vi "read Txt Files.vi"(10 "file path (use dialog)":path) -> (1 "error out":errorcluster, 2 "number":T1)   [LabVIEW 2017] (continued)
Voltage¡G\t0.005524\nReal Periold(ms)¡G\t1\tEncoder Position(0.1mm)¡G\t0.000000\tVelocity(0.1mm0/s)¡G\t0.000000\tVoltage¡G\t-0.016754\nReal Periold(ms)¡G\t1\tEncoder Position(0.1mm)¡G\t0.000000\tVelocity(0.1mm0/s)¡G\t0.000000\tVoltage¡G\t-0.003723\nReal Periold(ms)¡G\t1\tEncoder Position(0.1mm)¡G\t0.000000\tVelocity(0.1mm0/s)¡G\t0.000000\tVoltage¡G\t0.012512\nReal Periold(ms)¡G\t1\tEncoder Position(0.1mm)¡G\t0.000000\tVelocity(0.1mm0/s)¡G\t0.000000\tVoltage¡G\t0.006775\nReal Periold(ms)¡G\t1\tEncoder Position(0.1mm)¡G\t0.000000\tVelocity(0.1mm0/s)¡G\t0.000000\tVoltage¡G\t-0.003082\nReal Periold(ms)¡G\t1\tEncoder Position(0.1mm)¡G\t0.000000\tVelocity(0.1mm0/s)¡G\t0.000000\tVoltage¡G\t-0.003387\nReal Periold(ms)¡G\t1\tEncoder Position(0.1mm)¡G\t0.000000\tVelocity(0.1mm0/s)¡G\t0.000000\tVoltage¡G\t0.005524\nReal Periold(ms)¡G\t1\tEncoder Position(0.1mm)¡G\t0.000000\tVelocity(0.1mm0/s)¡G\t0.000000\tVoltage¡G\t-0.001160\nReal Periold(ms)¡G\t1\tEncoder Position(0.1mm)¡G\t0.000000\tVelocity(0.1mm0/s)¡G\t0.000000\tVoltage¡G\t-0.001495\nReal Periold(ms)¡G\t1\tEncoder Position(0.1mm)¡G\t0.000000\tVelocity(0.1mm0/s)¡G\t0.000000\tVoltage¡G\t0.001678\nReal Periold(ms)¡G\t1\tEncoder Position(0.1mm)¡G\t0.000000\tVelocity(0.1mm0/s)¡G\t0.000000\tVoltage¡G\t-0.014221\nReal Periold(ms)¡G\t1\tEncoder Position(0.1mm)¡G\t0.000000\tVelocity(0.1mm0/s)¡G\t0.000000\tVoltage¡G\t-0.005005\nReal Periold(ms)¡G\t1\tEncoder Position(0.1mm)¡G\t0.000000\tVelocity(0.1mm0/s)¡G\t0.000000\tVoltage¡G\t0.003906\nReal Periold(ms)¡G\t1\tEncoder Position(0.1mm)¡G\t0.000000\tVelocity(0.1mm0/s)¡G\t0.000000\tVoltage¡G\t-0.000214\nReal Periold(ms)¡G\t1\tEncoder Position(0.1mm)¡G\t0.000000\tVelocity(0.1mm0/s)¡G\t0.000000\tVoltage¡G\t0.001678\nReal Periold(ms)¡G\t1\tEncoder Position(0.1mm)¡G\t0.000000\tVelocity(0.1mm0/s)¡G\t0.000000\tVoltage¡G\t-0.009766\nReal Periold(ms)¡G\t1\tEncoder Position(0.1mm)¡G\t0.000000\tVelocity(0.1mm0/s)¡G\t0.000000\tVoltage¡G\t-0.021240\nReal Periold(ms)¡G\t1\tEncoder Position(0.1mm)¡G\t0.000000\tVelocity(0.1mm0/s)¡G\t0.000000\tVoltage¡G\t0.002319\nReal Periold(ms)¡G\t1\tEncoder Position(0.1mm)¡G\t0.000000\tVelocity(0.1mm0/s)¡G\t0.000000\tVoltage¡G\t-0.000854\nReal Periold(ms)¡G\t1\tEncoder Position(0.1mm)¡G\t0.000000\tVelocity(0.1mm0/s)¡G\t0.000000\tVoltage¡G\t0.006470\nReal Periold(ms)¡G\t1\tEncoder Position(0.1mm)¡G\t0.000000\tVelocity(0.1mm0/s)¡G\t0.000000\tVoltage¡G\t-0.002777\nReal Periold(ms)¡G\t1\tEncoder Position(0.1mm)¡G\t0.000000\tVelocity(0.1mm0/s)¡G\t0.000000\tVoltage¡G\t-0.004028\nReal Periold(ms)¡G\t1\tEncoder Position(0.1mm)¡G\t0.000000\tVelocity(0.1mm0/s)¡G\t0.000000\tVoltage¡G\t-0.016144\nReal Periold(ms)¡G\t1\tEncoder Position(0.1mm)¡G\t0.000000\tVelocity(0.1mm0/s)¡G\t0.000000\tVoltage¡G\t0.004547\nReal Periold(ms)¡G\t1\tEncoder Position(0.1mm)¡G\t0.000000\tVelocity(0.1mm0/s)¡G\t0.000000\tVoltage¡G\t-0.010071\nReal Periold(ms)¡G\t1\tEncoder Position(0.1mm)¡G\t0.000000\tVelocity(0.1mm0/s)¡G\t0.000000\tVoltage¡G\t-0.008179\nReal Periold(ms)¡G\t1\tEncoder Position(0.1mm)¡G\t0.000000\tVelocity(0.1mm0/s)¡G\t0.000000\tVoltage¡G\t-0.011047\nReal Periold(ms)¡G\t1\tEncoder Position(0.1mm)¡G\t0.000000\tVelocity(0.1mm0/s)¡G\t0.000000\tVoltage¡G\t-0.005951\nReal Periold(ms)¡G\t1\tEncoder Position(0.1mm)¡G\t0.000000\tVelocity(0.1mm0/s)¡G\t0.000000\tVoltage¡G\t0.002960\nReal Periold(ms)¡G\t1\tEncoder Position(0.1mm)¡G\t0.000000\tVelocity(0.1mm0/s)¡G\t0.000000\tVoltage¡G\t0.002960\nReal Periold(ms)¡G\t1\tEncoder Position(0.1mm)¡G\t0.000000\tVelocity(0.1mm0/s)¡G\t0.000000\tVoltage¡G\t0.007751\nReal Periold(ms)¡G\t1\tEncoder Position(0.1mm)¡G\t0.000000\tVelocity(0.1mm0/s)¡G\t0.000000\tVoltage¡G\t-0.003387\nReal Periold(ms)¡G\t1\tEncoder Position(0.1mm)¡G\t0.000000\tVelocity(0.1mm0/s)¡G\t0.000000\tVoltage¡G\t-0.005615\nReal Periold(ms)¡G\t1\tEncoder Position(0.1mm)¡G\t0.000000\tVelocity(0.1mm0/s)¡G\t0.000000\tVoltage¡G\t-0.002136\nReal Periold(ms)¡G\t1\tEncoder Position(0.1mm)¡G\t0.000000\tVelocity(0.1mm0/s)¡G\t0.000000\tVoltage¡G\t-0.002777\nReal Periold(ms)¡G\t1\tEncoder Position(0.1mm)¡G\t0.000000\tVelocity(0.1mm0/s)¡G\t0.000000\tVoltage¡G\t-0.007843\nReal Periold(ms)¡G\t1\tEncoder Position(0.1mm)¡G\t0.000000\tVelocity(0.1mm0/s)¡G\t0.000000\tVoltage¡G\t0.000732\nReal Periold(ms)¡G\t1\tEncoder Position(0.1mm)¡G\t0.000000\tVelocity(0.1mm0/s)¡G\t0.000000\tVoltage¡G\t-0.001495\nReal Periold(ms)¡G\t1\tEncoder Position(0.1mm)¡G\t0.000000\tVelocity(0.1mm0/s)¡G\t0.000000\tVoltage¡G\t-0.008179\nReal Periold(ms)¡G\t1\tEncoder Position(0.1mm)¡G\t0.000000\tVelocity(0.1mm0/s)¡G\t0.000000\tVoltage¡G\t-0.010406\nReal Periold(ms)¡G\t1\tEncoder Position(0.1mm)¡G\t0.000000\tVelocity(0.1mm0/s)¡G\t0.000000\tVoltage¡G\t-0.003723\nReal Periold(ms)¡G\t1\tEncoder Position(0.1mm)¡G\t0.000000\tVelocity(0.1mm0/s)¡G\t0.000000\tVoltage¡G\t0.002319\nReal Periold(ms)¡G\t1\tEncoder Position(0.1mm)¡G\t0.000000\tVelocity(0.1mm0/s)¡G\t0.000000\tVoltage¡G\t-0.001495\nReal Periold(ms)¡G\t1\tEncoder Position(0.1mm)¡G\t0.000000\tVelocity(0.1mm0/s)¡G\t0.000000\tVoltage¡G\t0.004242\nReal Periold(ms)¡G\t1\tEncoder Position(0.1mm)¡G\t0.000000\tVelocity(0.1mm0/s)¡G\t0.000000\tVoltage¡G\t0.011566\nReal Periold(ms)¡G\t1\tEncoder Position(0.1mm)¡G\t0.000000\tVelocity(0.1mm0/s)¡G\t0.000000\tVoltage¡G\t-0.000214\nReal Periold(ms)¡G\t1\tEncoder Position(0.1mm)¡G\t0.000000\tVelocity(0.1mm0/s)¡G\t0.000000\tVoltage¡G\t0.004242\nReal Periold(ms)¡G\t1\tEncoder Position(0.1mm)¡G\t0.000000\tVelocity(0.1mm0/s)¡G\t0.000000\tVoltage¡G\t-0.009125\nReal Periold(ms)¡G\t1\tEncoder Position(0.1mm)¡G\t0.000000\tVelocity(0.1mm0/s)¡G\t0.000000\tVoltage¡G\t-0.000854\nReal Periold(ms)¡G\t1\tEncoder Position(0.1mm)¡G\t0.000000\tVelocity(0.1mm0/s)¡G\t0.000000\tVoltage¡G\t-0.004669\nReal Periold(ms)¡G\t1\tEncoder Position(0.1mm)¡G\t0.000000\tVelocity(0.1mm0/s)¡G\t0.000000\tVoltage¡G\t0.005829\nReal Periold(ms)¡G\t1\tEncoder Position(0.1mm)¡G\t0.000000\tVelocity(0.1mm0/s)¡G\t0.000000\tVoltage¡G\t-0.013580\nReal Periold(ms)¡G\t1\tEncoder Position(0.1mm)¡G\t0.000000\tVelocity(0.1mm0/s)¡G\t0.000000\tVoltage¡G\t-0.005951\nReal Periold(ms)¡G\t1\tEncoder Position(0.1mm)¡G\t0.000000\tVelocity(0.1mm0/s)¡G\t0.000000\tVoltage¡G\t-0.002777\nReal Periold(ms)¡G\t1\tEncoder Position(0.1mm)¡G\t0.000000\tVelocity(0.1mm0/s)¡G\t0.000000\tVoltage¡G\t0.006470\nReal Periold(ms)¡G\t1\tEncoder Position(0.1mm)¡G\t0.000000\tVelocity(0.1mm0/s)¡G\t0.000000\tVoltage¡G\t0.000427\nReal Periold(ms)¡G\t1\tEncoder Position(0.1mm)¡G\t0.000000\tVelocity(0.1mm0/s)¡G\t0.000000\tVoltage¡G\t0.008362\nReal Periold(ms)¡G\t1\tEncoder Position(0.1mm)¡G\t0.000000\tVelocity(0.1mm0/s)¡G\t0.000000\tVoltage¡G\t0.000092\nReal Periold(ms)¡G\t1\tEncoder Position(0.1mm)¡G\t0.000000\tVelocity(0.1mm0/s)¡G\t0.000000\tVoltage¡G\t-0.004028\nReal Periold(ms)¡G\t1\tEncoder Position(0.1mm)¡G\t0.000000\tVelocity(0.1mm0/s)¡G\t0.000000\tVoltage¡G\t-0.004364\nReal Periold(ms)¡G\t1\tEncoder Position(0.1mm)¡G\t0.000000\tVelocity(0.1mm0/s)¡G\t0.000000\tVoltage¡G\t0.007111\nReal Periold(ms)¡G\t1\tEncoder Position(0.1mm)¡G\t0.000000\tVelocity(0.1mm0/s)¡G\t0.000000\tVoltage¡G\t-0.013916\nReal Periold(ms)¡G\t1\tEncoder Position(0.1mm)¡G\t0.000000\tVelocity(0.1mm0/s)¡G\t0.000000\tVoltage¡G\t0.000732\nReal Periold(ms)¡G\t1\tEncoder Position(0.1mm)¡G\t0.000000\tVelocity(0.1mm0/s)¡G\t0.000000\tVoltage¡G\t-0.009766\nReal Periold(ms)¡G\t1\tEncoder Position(0.1mm)¡G\t0.000000\tVelocity(0.1mm0/s)¡G\t0.000000\tVoltage¡G\t0.000092\nReal Periold(ms)¡G\t1\tEncoder Position(0.1mm)¡G\t0.000000\tVelocity(0.1mm0/s)¡G\t0.000000\tVoltage¡G\t0.002319\nReal Periold(ms)¡G\t1\tEncoder Position(0.1mm)¡G\t0.000000\tVelocity(0.1mm0/s)¡G\t0.000000\tVoltage¡G\t-0.005005\nReal Periold(ms)¡G\t1\tEncoder Position(0.1mm)¡G\t0.000000\tVelocity(0.1mm0/s)¡G\t0.000000\tVoltage¡G\t0.009003\nReal Periold(ms)¡G\t1\tEncoder Position(0.1mm)¡G\t0.000000\tVelocity(0.1mm0/s)¡G\t0.000000\tVoltage¡G\t0.014099\nReal Periold(ms)¡G\t1\tEncoder Position(0.1mm)¡G\t0.000000\tVelocity(0.1mm0/s)¡G\t0.000000\tVoltage¡G\t0.002960\nReal Periold(ms)¡G\t1\tEncoder Position(0.1mm)¡G\t0.000000\tVelocity(0.1mm0/s)¡G\t0.000000\tVoltage¡G\t0.000732\nReal Periold(ms)¡G\t1\tEncoder Position(0.1mm)¡G\t0.000000\tVelocity(0.1mm0/s)¡G\t0.000000\tVoltage¡G\t-0.005310\nReal Periold(ms)¡G\t1\tEncoder Position(0.1mm)¡G\t0.000000\tVelocity(0.1mm0/s)¡G\t0.000000\tVoltage¡G\t0.003906\nReal Periold(ms)¡G\t1\tEncoder Position(0.1mm)¡G\t0.000000\tVelocity(0.1mm0/s)¡G\t0.000000\tVoltage¡G\t-0.034271\nReal Periold(ms)¡G\t1\tEncoder Position(0.1mm)¡G\t0.000000\tVelocity(0.1mm0/s)¡G\t0.000000\tVoltage¡G\t-0.012634\nReal Periold(ms)¡G\t1\tEncoder Position(0.1mm)¡G\t0.000000\tVelocity(0.1mm0/s)¡G\t0.000000\tVoltage¡G\t-0.002136\nReal Periold(ms)¡G\t1\tEncoder Position(0.1mm)¡G\t0.000000\tVelocity(0.1mm0/s)¡G\t0.000000\tVoltage¡G\t0.009644\nReal Periold(ms)¡G\t1\tEncoder Position(0.1mm)¡G\t0.000000\tVelocity(0.1mm0/s)¡G\t0.000000\tVoltage¡G\t0.000092\nReal Periold(ms)¡G\t1\tEncoder Position(0.1mm)¡G\t0.000000\tVelocity(0.1mm0/s)¡G\t0.000000\tVoltage¡G\t0.000427\nReal Periold(ms)¡G\t1\tEncoder Position(0.1mm)¡G\t0.000000\tVelocity(0.1mm0/s)¡G\t0.000000\tVoltage¡G\t-0.002441\nReal Periold(ms)¡G\t1\tEncoder Position(0.1mm)¡G\t0.000000\tVelocity(0.1mm0/s)¡G\t0.000000\tVoltage¡G\t-0.006256\nReal Periold(ms)¡G\t1\tEncoder Position(0.1mm)¡G\t0.000000\tVelocity(0.1mm0/s)¡G\t0.000000\tVoltage¡G\t0.007751\nReal Periold(ms)¡G\t1\tEncoder Position(0.1mm)¡G\t0.000000\tVelocity(0.1mm0/s)¡G\t0.000000\tVoltage¡G\t0.000092\nReal Periold(ms)¡G\t1\tEncoder Position(0.1mm)¡G\t0.000000\tVelocity(0.1mm0/s)¡G\t0.000000\tVoltage¡G\t0.008698\nReal Periold(ms)¡G\t1\tEncoder Position(0.1mm)¡G\t0.000000\tVelocity(0.1mm0/s)¡G\t0.000000\tVoltage¡G\t0.010590\nReal Periold(ms)¡G\t1\tEncoder Position(0.1mm)¡G\t0.000000\tVelocity(0.1mm0/s)¡G\t0.000000\tVoltage¡G\t-0.002441\nReal Periold(ms)¡G\t1\tEncoder Position(0.1mm)¡G\t0.000000\tVelocity(0.1mm0/s)¡G\t0.000000\tVoltage¡G\t-0.008484\nReal Periold(ms)¡G\t1\tEncoder Position(0.1mm)¡G\t0.000000\tVelocity(0.1mm0/s)¡G\t0.000000\tVoltage¡G\t-0.001801\nReal Periold(ms)¡G\t1\tEncoder Position(0.1mm)¡G\t0.000000\tVelocity(0.1mm0/s)¡G\t0.000000\tVoltage¡G\t0.001373\nReal Periold(ms)¡G\t1\tEncoder Position(0.1mm)¡G\t0.000000\tVelocity(0.1mm0/s)¡G\t0.000000\tVoltage¡G\t-0.011993\nReal Periold(ms)¡G\t1\tEncoder Position(0.1mm)¡G\t0.000000\tVelocity(0.1mm0/s)¡G\t0.000000\tVoltage¡G\t-0.005615\nReal Periold(ms)¡G\t1\tEncoder Position(0.1mm)¡G\t0.000000\tVelocity(0.1mm0/s)¡G\t0.000000\tVoltage¡G\t0.014740\nReal Periold(ms)¡G\t1\tEncoder Position(0.1mm)¡G\t0.000000\tVelocity(0.1mm0/s)¡G\t0.000000\tVoltage¡G\t-0.000214\nReal Periold(ms)¡G\t1\tEncoder Position(0.1mm)¡G\t0.000000\tVelocity(0.1mm0/s)¡G\t0.000000\tVoltage¡G\t0.009979\nReal Periold(ms)¡G\t1\tEncoder Position(0.1mm)¡G\t0.000000\tVelocity(0.1mm0/s)¡G\t0.000000\tVoltage¡G\t-0.002441\nReal Periold(ms)¡G\t1\tEncoder Position(0.1mm)¡G\t0.000000\tVelocity(0.1mm0/s)¡G\t0.000000\tVoltage¡G\t-0.005005\nReal Periold(ms)¡G\t1\tEncoder Position(0.1mm)¡G\t0.000000\tVelocity(0.1mm0/s)¡G\t0.000000\tVoltage¡G\t0.003601\nReal Periold(ms)¡G\t1\tEncoder Position(0.1mm)¡G\t0.000000\tVelocity(0.1mm0/s)¡G\t0.000000\tVoltage¡G\t0.002960\nReal Periold(ms)¡G\t1\tEncoder Position(0.1mm)¡G\t0.000000\tVelocity(0.1mm0/s)¡G\t0.000000\tVoltage¡G\t0.003601\nReal Periold(ms)¡G\t1\tEncoder Position(0.1mm)¡G\t0.000000\tVelocity(0.1mm0/s)¡G\t0.000000\tVoltage¡G\t-0.007843\nReal Periold(ms)¡G\t1\tEncoder Position(0.1mm)¡G\t0.000000\tVelocity(0.1mm0/s)¡G\t0.000000\tVoltage¡G\t-0.001495\nReal Periold(ms)¡G\t1\tEncoder Position(0.1mm)¡G\t0.000000\tVelocity(0.1mm0/s)¡G\t0.000000\tVoltage¡G\t-0.001495\nReal Periold(ms)¡G\t1\tEncoder Position(0.1mm)¡G\t0.000000\tVelocity(0.1mm0/s)¡G\t0.000000\tVoltage¡G\t0.002319\nReal Periold(ms)¡G\t1\tEncoder Position(0.1mm)¡G\t0.000000\tVelocity(0.1mm0/s)¡G\t0.000000\tVoltage¡G\t0.006775\nReal Periold(ms)¡G\t1\tEncoder Position(0.1mm)¡G\t0.000000\tVelocity(0.1mm0/s)¡G\t0.000000\tVoltage¡G\t0.000092\nReal Periold(ms)¡G\t1\tEncoder Position(0.1mm)¡G\t0.000000\tVelocity(0.1mm0/s)¡G\t0.000000\tVoltage¡G\t0.006134\nReal Periold(ms)¡G\t1\tEncoder Position(0.1mm)¡G\t0.000000\tVelocity(0.1mm0/s)¡G\t0.000000\tVoltage¡G\t0.003906\nReal Periold(ms)¡G\t1\tEncoder Position(0.1mm)¡G\t0.000000\tVelocity(0.1mm0/s)¡G\t0.000000\tVoltage¡G\t0.004883\nReal Periold(ms)¡G\t1\tEncoder Position(0.1mm)¡G\t0.000000\tVelocity(0.1mm0/s)¡G\t0.000000\tVoltage¡G\t-0.002777\nReal Periold(ms)¡G\t1\tEncoder Position(0.1mm)¡G\t0.000000\tVelocity(0.1mm0/s)¡G\t0.000000\tVoltage¡G\t-0.007538\nReal Periold(ms)¡G\t1\tEncoder Position(0.1mm)¡G\t0.000000\tVelocity(0.1mm0/s)¡G\t0.000000\tVoltage¡G\t-0.003387\nReal Periold(ms)¡G\t1\tEncoder Position(0.1mm)¡G\t0.000000\tVelocity(0.1mm0/s)¡G\t0.000000\tVoltage¡G\t-0.014526\nReal Periold(ms)¡G\t1\tEncoder Position(0.1mm)¡G\t0.000000\tVelocity(0.1mm0/s)¡G\t0.000000\tVoltage¡G\t-0.004364\nReal Periold(ms)¡G\t1\tEncoder Position(0.1mm)¡G\t0.000000\tVelocity(0.1mm0/s)¡G\t0.000000\tVoltage¡G\t-0.000549\nReal Periold(ms)¡G\t1\tEncoder Position(0.1mm)¡G\t0.000000\tVelocity(0.1mm0/s)¡G\t0.000000\tVoltage¡G\t0.003296\nReal Periold(ms)¡G\t1\tEncoder Position(0.1mm)¡G\t0.000000\tVelocity(0.1mm0/s)¡G\t0.000000\tVoltage¡G\t-0.004028\nReal Periold(ms)¡G\t1\tEncoder Position(0.1mm)¡G\t0.000000\tVelocity(0.1mm0/s)¡G\t0.000000\tVoltage¡G\t0.002960\nReal Periold(ms)¡G\t1\tEncoder Position(0.1mm)¡G\t0.000000\tVelocity(0.1mm0/s)¡G\t0.000000\tVoltage¡G\t-0.006256\nReal Periold(ms)¡G\t1\tEncoder Position(0.1mm)¡G\t0.000000\tVelocity(0.1mm0/s)¡G\t0.000000\tVoltage¡G\t0.004242\nReal Periold(ms)¡G\t1\tEncoder Position(0.1mm)¡G\t0.000000\tVelocity(0.1mm0/s)¡G\t0.000000\tVoltage¡G\t-0.013916\nReal Periold(ms)¡G\t1\tEncoder Position(0.1mm)¡G\t0.000000\tVelocity(0.1mm0/s)¡G\t0.000000\tVoltage¡G\t0.005188\nReal Periold(ms)¡G\t1\tEncoder Position(0.1mm)¡G\t0.000000\tVelocity(0.1mm0/s)¡G\t0.000000\tVoltage¡G\t-0.015808\nReal Periold(ms)¡G\t1\tEncoder Position(0.1mm)¡G\t0.000000\tVelocity(0.1mm0/s)¡G\t0.000000\tVoltage¡G\t-0.007843\nReal Periold(ms)¡G\t1\tEncoder Position(0.1mm)¡G\t0.000000\tVelocity(0.1mm0/s)¡G\t0.000000\tVoltage¡G\t-0.005310\nReal Periold(ms)¡G\t1\tEncoder Position(0.1mm)¡G\t0.000000\tVelocity(0.1mm0/s)¡G\t0.000000\tVoltage¡G\t0.002960\nReal Periold(ms)¡G\t1\tEncoder Position(0.1mm)¡G\t0.000000\tVelocity(0.1mm0/s)¡G\t0.000000\tVoltage¡G\t-0.006256\nReal Periold(ms)¡G\t1\tEncoder Position(0.1mm)¡G\t0.000000\tVelocity(0.1mm0/s)¡G\t0.000000\tVoltage¡G\t0.001678\nReal Periold(ms)¡G\t1\tEncoder Position(0.1mm)¡G\t0.000000\tVelocity(0.1mm0/s)¡G\t0.000000\tVoltage¡G\t-0.013916\nReal Periold(ms)¡G\t1\tEncoder Position(0.1mm)¡G\t0.000000\tVelocity(0.1mm0/s)¡G\t0.000000\tVoltage¡G\t0.007751\nReal Periold(ms)¡G\t1\tEncoder Position(0.1mm)¡G\t0.000000\tVelocity(0.1mm0/s)¡G\t0.000000\tVoltage¡G\t0.009338\nReal Periold(ms)¡G\t1\tEncoder Position(0.1mm)¡G\t0.000000\tVelocity(0.1mm0/s)¡G\t0.000000\tVoltage¡G\t-0.002136\nReal Periold(ms)¡G\t1\tEncoder Position(0.1mm)¡G\t0.000000\tVelocity(0.1mm0/s)¡G\t0.000000\tVoltage¡G\t0.002014\nReal Periold(ms)¡G\t1\tEncoder Position(0.1mm)¡G\t0.000000\tVelocity(0.1mm0/s)¡G\t0.000000\tVoltage¡G\t0.002319\nReal Periold(ms)¡G\t1\tEncoder Position(0.1mm)¡G\t0.000000\tVelocity(0.1mm0/s)¡G\t0.000000\tVoltage¡G\t-0.009125\nReal Periold(ms)¡G\t1\tEncoder Position(0.1mm)¡G\t0.000000\tVelocity(0.1mm0/s)¡G\t0.000000\tVoltage¡G\t0.001068\nReal Periold(ms)¡G\t1\tEncoder Position(0.1mm)¡G\t0.000000\tVelocity(0.1mm0/s)¡G\t0.000000\tVoltage¡G\t-0.011993\nReal Periold(ms)¡G\t1\tEncoder Position(0.1mm)¡G\t0.000000\tVelocity(0.1mm0/s)¡G\t0.000000\tVoltage¡G\t0.006470\nReal Periold(ms)¡G\t1\tEncoder Position(0.1mm)¡G\t0.000000\tVelocity(0.1mm0/s)¡G\t0.000000\tVoltage¡G\t-0.002136\nReal Periold(ms)¡G\t1\tEncoder Position(0.1mm)¡G\t0.000000\tVelocity(0.1mm0/s)¡G\t0.000000\tVoltage¡G\t-0.006592\nReal Periold(ms)¡G\t1\tEncoder Position(0.1mm)¡G\t0.000000\tVelocity(0.1mm0/s)¡G\t0.000000\tVoltage¡G\t-0.004364\nReal Periold(ms)¡G\t1\tEncoder Position(0.1mm)¡G\t0.000000\tVelocity(0.1mm0/s)¡G\t0.000000\tVoltage¡G\t0.000732\nReal Periold(ms)¡G\t1\tEncoder Position(0.1mm)¡G\t0.000000\tVelocity(0.1mm0/s)¡G\t0.000000\tVoltage¡G\t-0.012299\nReal Periold(ms)¡G\t1\tEncoder Position(0.1mm)¡G\t0.000000\tVelocity(0.1mm0/s)¡G\t0.000000\tVoltage¡G\t-0.000549\nReal Periold(ms)¡G\t1\tEncoder Position(0.1mm)¡G\t0.000000\tVelocity(0.1mm0/s)¡G\t0.000000\tVoltage¡G\t-0.006256\nReal Periold(ms)¡G\t1\tEncoder Position(0.1mm)¡G\t0.000000\tVelocity(0.1mm0/s)¡G\t0.000000\tVoltage¡G\t0.001373\nReal Periold(ms)¡G\t1\tEncoder Position(0.1mm)¡G\t0.000000\tVelocity(0.1mm0/s)¡G\t0.000000\tVoltage¡G\t0.004883\nReal Periold(ms)¡G\t1\tEncoder Position(0.1mm)¡G\t0.000000\tVelocity(0.1mm0/s)¡G\t0.000000\tVoltage¡G\t0.006134\nReal Periold(ms)¡G\t1\tEncoder Position(0.1mm)¡G\t0.000000\tVelocity(0.1mm0/s)¡G\t0.000000\tVoltage¡G\t-0.005615\nReal Periold(ms)¡G\t1\tEncoder Position(0.1mm)¡G\t0.000000\tVelocity(0.1mm0/s)¡G\t0.000000\tVoltage¡G\t0.003296\nReal Periold(ms)¡G\t1\tEncoder Position(0.1mm)¡G\t0.000000\tVelocity(0.1mm0/s)¡G\t0.000000\tVoltage¡G\t-0.003387\nReal Periold(ms)¡G\t1\tEncoder Position(0.1mm)¡G\t0.000000\tVelocity(0.1mm0/s)¡G\t0.000000\tVoltage¡G\t-0.012939\nReal Periold(ms)¡G\t1\tEncoder Position(0.1mm)¡G\t0.000000\tVelocity(0.1mm0/s)¡G\t0.000000\tVoltage¡G\t0.014740\nReal Periold(ms)¡G\t1\tEncoder Position(0.1mm)¡G\t0.000000\tVelocity(0.1mm0/s)¡G\t0.000000\tVoltage¡G\t-0.008179\nReal Periold(ms)¡G\t1\tEncoder Position(0.1mm)¡G\t0.000000\tVelocity(0.1mm0/s)¡G\t0.000000\tVoltage¡G\t-0.002441\nReal Periold(ms)¡G\t1\tEncoder Position(0.1mm)¡G\t0.000000\tVelocity(0.1mm0/s)¡G\t0.000000\tVoltage¡G\t-0.004364\nReal Periold(ms)¡G\t1\tEncoder Position(0.1mm)¡G\t0.000000\tVelocity(0.1mm0/s)¡G\t0.000000\tVoltage¡G\t0.002319\nReal Periold(ms)¡G\t1\tEncoder Position(0.1mm)¡G\t0.000000\tVelocity(0.1mm0/s)¡G\t0.000000\tVoltage¡G\t-0.003723\nReal Periold(ms)¡G\t1\tEncoder Position(0.1mm)¡G\t0.000000\tVelocity(0.1mm0/s)¡G\t0.000000\tVoltage¡G\t0.018890\nReal Periold(ms)¡G\t1\tEncoder Position(0.1mm)¡G\t0.000000\tVelocity(0.1mm0/s)¡G\t0.000000\tVoltage¡G\t0.007111\nReal Periold(ms)¡G\t1\tEncoder Position(0.1mm)¡G\t0.000000\tVelocity(0.1mm0/s)¡G\t0.000000\tVoltage¡G\t0.020782\nReal Periold(ms)¡G\t1\tEncoder Position(0.1mm)¡G\t0.000000\tVelocity(0.1mm0/s)¡G\t0.000000\tVoltage¡G\t-0.002136\nReal Periold(ms)¡G\t1\tEncoder Position(0.1mm)¡G\t0.000000\tVelocity(0.1mm0/s)¡G\t0.000000\tVoltage¡G\t0.003296\nReal Periold(ms)¡G\t1\tEncoder Position(0.1mm)¡G\t0.000000\tVelocity(0.1mm0/s)¡G\t0.000000\tVoltage¡G\t-0.010406\nReal Periold(ms)¡G\t1\tEncoder Position(0.1mm)¡G\t0.000000\tVelocity(0.1mm0/s)¡G\t0.000000\tVoltage¡G\t0.000092\nReal Periold(ms)¡G\t1\tEncoder Position(0.1mm)¡G\t0.000000\tVelocity(0.1mm0/s)¡G\t0.000000\tVoltage¡G\t-0.021240\nReal Periold(ms)¡G\t1\tEncoder Position(0.1mm)¡G\t0.000000\tVelocity(0.1mm0/s)¡G\t0.000000\tVoltage¡G\t-0.017731\nReal Periold(ms)¡G\t1\tEncoder Position(0.1mm)¡G\t0.000000\tVelocity(0.1mm0/s)¡G\t0.000000\tVoltage¡G\t-0.013275\nReal Periold(ms)¡G\t1\tEncoder Position(0.1mm)¡G\t0.000000\tVelocity(0.1mm0/s)¡G\t0.000000\tVoltage¡G\t-0.000214\nReal Periold(ms)¡G\t1\tEncoder Position(0.1mm)¡G\t0.000000\tVelocity(0.1mm0/s)¡G\t0.000000\tVoltage¡G\t-0.010071\nReal Periold(ms)¡G\t1\tEncoder Position(0.1mm)¡G\t0.000000\tVelocity(0.1mm0/s)¡G\t0.000000\tVoltage¡G\t-0.008179\nReal Periold(ms)¡G\t1\tEncoder Position(0.1mm)¡G\t0.000000\tVelocity(0.1mm0/s)¡G\t0.000000\tVoltage¡G\t-0.005615\nReal Periold(ms)¡G\t1\tEncoder Position(0.1mm)¡G\t0.000000\tVelocity(0.1mm0/s)¡G\t0.000000\tVoltage¡G\t-0.003723\nReal Periold(ms)¡G\t1\tEncoder Position(0.1mm)¡G\t0.000000\tVelocity(0.1mm0/s)¡G\t0.000000\tVoltage¡G\t-0.001160\nReal Periold(ms)¡G\t1\tEncoder Position(0.1mm)¡G\t0.000000\tVelocity(0.1mm0/s)¡G\t0.000000\tVoltage¡G\t0.003906\nReal Periold(ms)¡G\t1\tEncoder Position(0.1mm)¡G\t0.000000\tVelocity(0.1mm0/s)¡G\t0.000000\tVoltage¡G\t0.007111\nReal Periold(ms)¡G\t1\tEncoder Position(0.1mm)¡G\t0.000000\tVelocity(0.1mm0/s)¡G\t0.000000\tVoltage¡G\t-0.003082\nReal Periold(ms)¡G\t1\tEncoder Position(0.1mm)¡G\t0.000000\tVelocity(0.1mm0/s)¡G\t0.000000\tVoltage¡G\t-0.014221\nReal Periold(ms)¡G\t1\tEncoder Position(0.1mm)¡G\t0.000000\tVelocity(0.1mm0/s)¡G\t0.000000\tVoltage¡G\t-0.004364\nReal Periold(ms)¡G\t1\tEncoder Position(0.1mm)¡G\t0.000000\tVelocity(0.1mm0/s)¡G\t0.000000\tVoltage¡G\t0.000732\nReal Periold(ms)¡G\t1\tEncoder Position(0.1mm)¡G\t0.000000\tVelocity(0.1mm0/s)¡G\t0.000000\tVoltage¡G\t-0.016754\nReal Periold(ms)¡G\t1\tEncoder Position(0.1mm)¡G\t0.000000\tVelocity(0.1mm0/s)¡G\t0.000000\tVoltage¡G\t-0.014526\nReal Periold(ms)¡G\t1\tEncoder Position(0.1mm)¡G\t0.000000\tVelocity(0.1mm0/s)¡G\t0.000000\tVoltage¡G\t-0.012939\nReal Periold(ms)¡G\t1\tEncoder Position(0.1mm)¡G\t0.000000\tVelocity(0.1mm0/s)¡G\t0.000000\tVoltage¡G\t0.011566\nReal Periold(ms)¡G\t1\tEncoder Position(0.1mm)¡G\t0.000000\tVelocity(0.1mm0/s)¡G\t0.000000\tVoltage¡G\t0.017273\nReal Periold(ms)¡G\t1\tEncoder Position(0.1mm)¡G\t0.000000\tVelocity(0.1mm0/s)¡G\t0.000000\tVoltage¡G\t-0.004028\nReal Periold(ms)¡G\t1\tEncoder Position(0.1mm)¡G\t0.000000\tVelocity(0.1mm0/s)¡G\t0.000000\tVoltage¡G\t-0.006256\nReal Periold(ms)¡G\t1\tEncoder Position(0.1mm)¡G\t0.000000\tVelocity(0.1mm0/s)¡G\t0.000000\tVoltage¡G\t-0.004364\nReal Periold(ms)¡G\t1\tEncoder Position(0.1mm)¡G\t0.000000\tVelocity(0.1mm0/s)¡G\t0.000000\tVoltage¡G\t-0.011993\nReal Periold(ms)¡G\t1\tEncoder Position(0.1mm)¡G\t0.000000\tVelocity(0.1mm0/s)¡G\t0.000000\tVoltage¡G\t0.001373\nReal Periold(ms)¡G\t1\tEncoder Position(0.1mm)¡G\t0.000000\tVelocity(0.1mm0/s)¡G\t0.000000\tVoltage¡G\t-0.005951\nReal Periold(ms)¡G\t1\tEncoder Position(0.1mm)¡G\t0.000000\tVelocity(0.1mm0/s)¡G\t0.000000\tVoltage¡G\t-0.000214\nReal Periold(ms)¡G\t1\tEncoder Position(0.1mm)¡G\t0.000000\tVelocity(0.1mm0/s)¡G\t0.000000\tVoltage¡G\t-0.004364\nReal Periold(ms)¡G\t1\tEncoder Position(0.1mm)¡G\t0.000000\tVelocity(0.1mm0/s)¡G\t0.000000\tVoltage¡G\t-0.003723\nReal Periold(ms)¡G\t1\tEncoder Position(0.1mm)¡G\t0.000000\tVelocity(0.1mm0/s)¡G\t0.000000\tVoltage¡G\t0.006775\nReal Periold(ms)¡G\t1\tEncoder Position(0.1mm)¡G\t0.000000\tVelocity(0.1mm0/s)¡G\t0.000000\tVoltage¡G\t-0.002777\nReal Periold(ms)¡G\t1\tEncoder Position(0.1mm)¡G\t0.000000\tVelocity(0.1mm0/s)¡G\t0.000000\tVoltage¡G\t-0.007538\nReal Periold(ms)¡G\t1\tEncoder Position(0.1mm)¡G\t0.000000\tVelocity(0.1mm0/s)¡G\t0.000000\tVoltage¡G\t-0.049561\nReal Periold(ms)¡G\t1\tEncoder Position(0.1mm)¡G\t0.000000\tVelocity(0.1mm0/s)¡G\t0.000000\tVoltage¡G\t0.003296\nReal Periold(ms)¡G\t1\tEncoder Position(0.1mm)¡G\t0.000000\tVelocity(0.1mm0/s)¡G\t0.000000\tVoltage¡G\t-0.000214\nReal Periold(ms)¡G\t1\tEncoder Position(0.1mm)¡G\t0.000000\tVelocity(0.1mm0/s)¡G\t0.000000\tVoltage¡G\t-0.004669\nReal Periold(ms)¡G\t1\tEncoder Position(0.1mm)¡G\t0.000000\tVelocity(0.1mm0/s)¡G\t0.000000\tVoltage¡G\t0.002960\nReal Periold(ms)¡G\t1\tEncoder Position(0.1mm)¡G\t0.000000\tVelocity(0.1mm0/s)¡G\t0.000000\tVoltage¡G\t-0.005615\nReal Periold(ms)¡G\t1\tEncoder Position(0.1mm)¡G\t0.000000\tVelocity(0.1mm0/s)¡G\t0.000000\tVoltage¡G\t-0.018677\nReal Periold(ms)¡G\t1\tEncoder Position(0.1mm)¡G\t0.000000\tVelocity(0.1mm0/s)¡G\t0.000000\tVoltage¡G\t-0.003387\nReal Periold(ms)¡G\t1\tEncoder Position(0.1mm)¡G\t0.000000\tVelocity(0.1mm0/s)¡G\t0.000000\tVoltage¡G\t-0.004364\nReal Periold(ms)¡G\t1\tEncoder Position(0.1mm)¡G\t0.000000\tVelocity(0.1mm0/s)¡G\t0.000000\tVoltage¡G\t0.000427\nReal Periold(ms)¡G\t1\tEncoder Position(0.1mm)¡G\t0.000000\tVelocity(0.1mm0/s)¡G\t0.000000\tVoltage¡G\t0.006775\nReal Periold(ms)¡G\t1\tEncoder Position(0.1mm)¡G\t0.000000\tVelocity(0.1mm0/s)¡G\t0.000000\tVoltage¡G\t0.001373\nReal Periold(ms)¡G\t1\tEncoder Position(0.1mm)¡G\t0.000000\tVelocity(0.1mm0/s)¡G\t0.000000\tVoltage¡G\t0.007111\nReal Periold(ms)¡G\t1\tEncoder Position(0.1mm)¡G\t0.000000\tVelocity(0.1mm0/s)¡G\t0.000000\tVoltage¡G\t0.003601\nReal Periold(ms)¡G\t1\tEncoder Position(0.1mm)¡G\t0.000000\tVelocity(0.1mm0/s)¡G\t0.000000\tVoltage¡G\t0.005524\nReal Periold(ms)¡G\t1\tEncoder Position(0.1mm)¡G\t0.000000\tVelocity(0.1mm0/s)¡G\t0.000000\tVoltage¡G\t-0.005951\nReal Periold(ms)¡G\t1\tEncoder Position(0.1mm)¡G\t0.000000\tVelocity(0.1mm0/s)¡G\t0.000000\tVoltage¡G\t0.010284\nReal Periold(ms)¡G\t1\tEncoder Position(0.1mm)¡G\t0.000000\tVelocity(0.1mm0/s)¡G\t0.000000\tVoltage¡G\t-0.006256\nReal Periold(ms)¡G\t1\tEncoder Position(0.1mm)¡G\t0.000000\tVelocity(0.1mm0/s)¡G\t0.000000\tVoltage¡G\t-0.003723\nReal Periold(ms)¡G\t1\tEncoder Position(0.1mm)¡G\t0.000000\tVelocity(0.1mm0/s)¡G\t0.000000\tVoltage¡G\t-0.012634\nReal Periold(ms)¡G\t1\tEncoder Position(0.1mm)¡G\t0.000000\tVelocity(0.1mm0/s)¡G\t0.000000\tVoltage¡G\t-0.002777\nReal Periold(ms)¡G\t1\tEncoder Position(0.1mm)¡G\t0.000000\tVelocity(0.1mm0/s)¡G\t0.000000\tVoltage¡G\t-0.005951\nReal Periold(ms)¡G\t1\tEncoder Position(0.1mm)¡G\t0.000000\tVelocity(0.1mm0/s)¡G\t0.000000\tVoltage¡G\t-0.002441\nReal Periold(ms)¡G\t1\tEncoder Position(0.1mm)¡G\t0.000000\tVelocity(0.1mm0/s)¡G\t0.000000\tVoltage¡G\t-0.063873\nReal Periold(ms)¡G\t1\tEncoder Position(0.1mm)¡G\t0.000000\tVelocity(0.1mm0/s)¡G\t0.000000\tVoltage¡G\t0.001678\nReal Periold(ms)¡G\t1\tEncoder Position(0.1mm)¡G\t0.000000\tVelocity(0.1mm0/s)¡G\t0.000000\tVoltage¡G\t-0.000549\nReal Periold(ms)¡G\t1\tEncoder Position(0.1mm)¡G\t0.000000\tVelocity(0.1mm0/s)¡G\t0.000000\tVoltage¡G\t0.003601\nReal Periold(ms)¡G\t1\tEncoder Position(0.1mm)¡G\t0.000000\tVelocity(0.1mm0/s)¡G\t0.000000\tVoltage¡G\t-0.000854\nReal Periold(ms)¡G\t1\tEncoder Position(0.1mm)¡G\t0.000000\tVelocity(0.1mm0/s)¡G\t0.000000\tVoltage¡G\t-0.001160\nReal Periold(ms)¡G\t1\tEncoder Position(0.1mm)¡G\t0.000000\tVelocity(0.1mm0/s)¡G\t0.000000\tVoltage¡G\t-0.004028\nReal Periold(ms)¡G\t1\tEncoder Position(0.1mm)¡G\t0.000000\tVelocity(0.1mm0/s)¡G\t0.000000\tVoltage¡G\t-0.000854\nReal Periold(ms)¡G\t1\tEncoder Position(0.1mm)¡G\t0.000000\tVelocity(0.1mm0/s)¡G\t0.000000\tVoltage¡G\t0.006470\nReal Periold(ms)¡G\t1\tEncoder Position(0.1mm)¡G\t0.000000\tVelocity(0.1mm0/s)¡G\t0.000000\tVoltage¡G\t0.001678\nReal Periold(ms)¡G\t1\tEncoder Position(0.1mm)¡G\t0.000000\tVelocity(0.1mm0/s)¡G\t0.000000\tVoltage¡G\t-0.005951\nReal Periold(ms)¡G\t1\tEncoder Position(0.1mm)¡G\t0.000000\tVelocity(0.1mm0/s)¡G\t0.000000\tVoltage¡G\t-0.005005\nReal Periold(ms)¡G\t1\tEncoder Position(0.1mm)¡G\t0.000000\tVelocity(0.1mm0/s)¡G\t0.000000\tVoltage¡G\t-0.002777\nReal Periold(ms)¡G\t1\tEncoder Position(0.1mm)¡G\t0.000000\tVelocity(0.1mm0/s)¡G\t0.000000\tVoltage¡G\t0.010284\nReal Periold(ms)¡G\t1\tEncoder Position(0.1mm)¡G\t0.000000\tVelocity(0.1mm0/s)¡G\t0.000000\tVoltage¡G\t0.000092\nReal Periold(ms)¡G\t1\tEncoder Position(0.1mm)¡G\t0.000000\tVelocity(0.1mm0/s)¡G\t0.000000\tVoltage¡G\t0.010590\nReal Periold(ms)¡G\t1\tEncoder Position(0.1mm)¡G\t0.000000\tVelocity(0.1mm0/s)¡G\t0.000000\tVoltage¡G\t0.007111\nReal Periold(ms)¡G\t1\tEncoder Position(0.1mm)¡G\t0.000000\tVelocity(0.1mm0/s)¡G\t0.000000\tVoltage¡G\t-0.004364\nReal Periold(ms)¡G\t1\tEncoder Position(0.1mm)¡G\t0.000000\tVelocity(0.1mm0/s)¡G\t0.000000\tVoltage¡G\t-0.002136\nReal Periold(ms)¡G\t1\tEncoder Position(0.1mm)¡G\t0.000000\tVelocity(0.1mm0/s)¡G\t0.000000\tVoltage¡G\t0.000427\nReal Periold(ms)¡G\t1\tEncoder Position(0.1mm)¡G\t0.000000\tVelocity(0.1mm0/s)¡G\t0.000000\tVoltage¡G\t-0.012634\nReal Periold(ms)¡G\t1\tEncoder Position(0.1mm)¡G\t0.000000\tVelocity(0.1mm0/s)¡G\t0.000000\tVoltage¡G\t0.003601\nReal Periold(ms)¡G\t1\tEncoder Position(0.1mm)¡G\t0.000000\tVelocity(0.1mm0/s)¡G\t0.000000\tVoltage¡G\t0.049744\nReal Periold(ms)¡G\t1\tEncoder Position(0.1mm)¡G\t0.000000\tVelocity(0.1mm0/s)¡G\t0.000000\tVoltage¡G\t0.009979\nReal Periold(ms)¡G\t1\tEncoder Position(0.1mm)¡G\t0.000000\tVelocity(0.1mm0/s)¡G\t0.000000\tVoltage¡G\t0.000732\nReal Periold(ms)¡G\t1\tEncoder Position(0.1mm)¡G\t0.000000\tVelocity(0.1mm0/s)¡G\t0.000000\tVoltage¡G\t0.003906\nReal Periold(ms)¡G\t1\tEncoder Position(0.1mm)¡G\t0.000000\tVelocity(0.1mm0/s)¡G\t0.000000\tVoltage¡G\t0.002655\nReal Periold(ms)¡G\t1\tEncoder Position(0.1mm)¡G\t0.000000\tVelocity(0.1mm0/s)¡G\t0.000000\tVoltage¡G\t-0.004364\nReal Periold(ms)¡G\t1\tEncoder Position(0.1mm)¡G\t0.000000\tVelocity(0.1mm0/s)¡G\t0.000000\tVoltage¡G\t-0.000214\nReal Periold(ms)¡G\t1\tEncoder Position(0.1mm)¡G\t0.000000\tVelocity(0.1mm0/s)¡G\t0.000000\tVoltage¡G\t-0.009125\nReal Periold(ms)¡G\t1\tEncoder Position(0.1mm)¡G\t0.000000\tVelocity(0.1mm0/s)¡G\t0.000000\tVoltage¡G\t-0.015503\nReal Periold(ms)¡G\t1\tEncoder Position(0.1mm)¡G\t0.000000\tVelocity(0.1mm0/s)¡G\t0.000000\tVoltage¡G\t0.007416\nReal Periold(ms)¡G\t1\tEncoder Position(0.1mm)¡G\t0.000000\tVelocity(0.1mm0/s)¡G\t0.000000\tVoltage¡G\t-0.005951\nReal Periold(ms)¡G\t1\tEncoder Position(0.1mm)¡G\t0.000000\tVelocity(0.1mm0/s)¡G\t0.000000\tVoltage¡G\t0.004547\nReal Periold(ms)¡G\t1\tEncoder Position(0.1mm)¡G\t0.000000\tVelocity(0.1mm0/s)¡G\t0.000000\tVoltage¡G\t-0.004669\nReal Periold(ms)¡G\t1\tEncoder Position(0.1mm)¡G\t0.000000\tVelocity(0.1mm0/s)¡G\t0.000000\tVoltage¡G\t-0.001160\nReal Periold(ms)¡G\t1\tEncoder Position(0.1mm)¡G\t0.000000\tVelocity(0.1mm0/s)¡G\t0.000000\tVoltage¡G\t-0.011047\nReal Periold(ms)¡G\t1\tEncoder Position(0.1mm)¡G\t0.000000\tVelocity(0.1mm0/s)¡G\t0.000000\tVoltage¡G\t-0.011688\nReal Periold(ms)¡G\t1\tEncoder Position(0.1mm)¡G\t0.000000\tVelocity(0.1mm0/s)¡G\t0.000000\tVoltage¡G\t0.006775\nReal Periold(ms)¡G\t1\tEncoder Position(0.1mm)¡G\t0.000000\tVelocity(0.1mm0/s)¡G\t0.000000\tVoltage¡G\t0.001678\nReal Periold(ms)¡G\t1\tEncoder Position(0.1mm)¡G\t0.000000\tVelocity(0.1mm0/s)¡G\t0.000000\tVoltage¡G\t-0.006592\nReal Periold(ms)¡G\t1\tEncoder Position(0.1mm)¡G\t0.000000\tVelocity(0.1mm0/s)¡G\t0.000000\tVoltage¡G\t-0.006897\nReal Periold(ms)¡G\t1\tEncoder Position(0.1mm)¡G\t0.000000\tVelocity(0.1mm0/s)¡G\t0.000000\tVoltage¡G\t-0.004364\nReal Periold(ms)¡G\t1\tEncoder Position(0.1mm)¡G\t0.000000\tVelocity(0.1mm0/s)¡G\t0.000000\tVoltage¡G\t-0.000214\nReal Periold(ms)¡G\t1\tEncoder Position(0.1mm)¡G\t0.000000\tVelocity(0.1mm0/s)¡G\t0.000000\tVoltage¡G\t-0.004364\nReal Periold(ms)¡G\t1\tEncoder Position(0.1mm)¡G\t0.000000\tVelocity(0.1mm0/s)¡G\t0.000000\tVoltage¡G\t0.014099\nReal Periold(ms)¡G\t1\tEncoder Position(0.1mm)¡G\t0.000000\tVelocity(0.1mm0/s)¡G\t0.000000\tVoltage¡G\t-0.008179\nReal Periold(ms)¡G\t1\tEncoder Position(0.1mm)¡G\t0.000000\tVelocity(0.1mm0/s)¡G\t0.000000\tVoltage¡G\t-0.010712\nReal Periold(ms)¡G\t1\tEncoder Position(0.1mm)¡G\t0.000000\tVelocity(0.1mm0/s)¡G\t0.000000\tVoltage¡G\t0.001373\nReal Periold(ms)¡G\t1\tEncoder Position(0.1mm)¡G\t0.000000\tVelocity(0.1mm0/s)¡G\t0.000000\tVoltage¡G\t-0.004364\nReal Periold(ms)¡G\t1\tEncoder Position(0.1mm)¡G\t0.000000\tVelocity(0.1mm0/s)¡G\t0.000000\tVoltage¡G\t0.001068\nReal Periold(ms)¡G\t1\tEncoder Position(0.1mm)¡G\t0.000000\tVelocity(0.1mm0/s)¡G\t0.000000\tVoltage¡G\t-0.009460\nReal Periold(ms)¡G\t1\tEncoder Position(0.1mm)¡G\t0.000000\tVelocity(0.1mm0/s)¡G\t0.000000\tVoltage¡G\t0.004242\nReal Periold(ms)¡G\t1\tEncoder Position(0.1mm)¡G\t0.000000\tVelocity(0.1mm0/s)¡G\t0.000000\tVoltage¡G\t-0.004028\nReal Periold(ms)¡G\t1\tEncoder Position(0.1mm)¡G\t0.000000\tVelocity(0.1mm0/s)¡G\t0.000000\tVoltage¡G\t0.000732\nReal Periold(ms)¡G\t1\tEncoder Position(0.1mm)¡G\t0.000000\tVelocity(0.1mm0/s)¡G\t0.000000\tVoltage¡G\t0.000092\nReal Periold(ms)¡G\t1\tEncoder Position(0.1mm)¡G\t0.000000\tVelocity(0.1mm0/s)¡G\t0.000000\tVoltage¡G\t-0.003082\nReal Periold(ms)¡G\t1\tEncoder Position(0.1mm)¡G\t0.000000\tVelocity(0.1mm0/s)¡G\t0.000000\tVoltage¡G\t0.037964\nReal Periold(ms)¡G\t1\tEncoder Position(0.1mm)¡G\t0.000000\tVelocity(0.1mm0/s)¡G\t0.000000\tVoltage¡G\t-0.007538\nReal Periold(ms)¡G\t1\tEncoder Position(0.1mm)¡G\t0.000000\tVelocity(0.1mm0/s)¡G\t0.000000\tVoltage¡G\t-0.003082\nReal Periold(ms)¡G\t1\tEncoder Position(0.1mm)¡G\t0.000000\tVelocity(0.1mm0/s)¡G\t0.000000\tVoltage¡G\t-0.014862\nReal Periold(ms)¡G\t1\tEncoder Position(0.1mm)¡G\t0.000000\tVelocity(0.1mm0/s)¡G\t0.000000\tVoltage¡G\t-0.006256\nReal Periold(ms)¡G\t1\tEncoder Position(0.1mm)¡G\t0.000000\tVelocity(0.1mm0/s)¡G\t0.000000\tVoltage¡G\t-0.000854\nReal Periold(ms)¡G\t1\tEncoder Position(0.1mm)¡G\t0.000000\tVelocity(0.1mm0/s)¡G\t0.000000\tVoltage¡G\t0.003296\nReal Periold(ms)¡G\t1\tEncoder Position(0.1mm)¡G\t0.000000\tVelocity(0.1mm0/s)¡G\t0.000000\tVoltage¡G\t-0.003387\nReal Periold(ms)¡G\t1\tEncoder Position(0.1mm)¡G\t0.000000\tVelocity(0.1mm0/s)¡G\t0.000000\tVoltage¡G\t0.005829\nReal Periold(ms)¡G\t1\tEncoder Position(0.1mm)¡G\t0.000000\tVelocity(0.1mm0/s)¡G\t0.000000\tVoltage¡G\t-0.010406\nReal Periold(ms)¡G\t1\tEncoder Position(0.1mm)¡G\t0.000000\tVelocity(0.1mm0/s)¡G\t0.000000\tVoltage¡G\t0.023346\nReal Periold(ms)¡G\t1\tEncoder Position(0.1mm)¡G\t0.000000\tVelocity(0.1mm0/s)¡G\t0.000000\tVoltage¡G\t0.070129\nReal Periold(ms)¡G\t1\tEncoder Position(0.1mm)¡G\t0.000000\tVelocity(0.1mm0/s)¡G\t0.000000\tVoltage¡G\t-0.005310\nReal Periold(ms)¡G\t1\tEncoder Position(0.1mm)¡G\t0.000000\tVelocity(0.1mm0/s)¡G\t0.000000\tVoltage¡G\t0.000732\nReal Periold(ms)¡G\t1\tEncoder Position(0.1mm)¡G\t0.000000\tVelocity(0.1mm0/s)¡G\t0.000000\tVoltage¡G\t0.001068\nReal Periold(ms)¡G\t1\tEncoder Position(0.1mm)¡G\t0.000000\tVelocity(0.1mm0/s)¡G\t0.000000\tVoltage¡G\t0.000732\nReal Periold(ms)¡G\t1\tEncoder Position(0.1mm)¡G\t0.000000\tVelocity(0.1mm0/s)¡G\t0.000000\tVoltage¡G\t-0.002441\nReal Periold(ms)¡G\t1\tEncoder Position(0.1mm)¡G\t0.000000\tVelocity(0.1mm0/s)¡G\t0.000000\tVoltage¡G\t-0.010071\nReal Periold(ms)¡G\t1\tEncoder Position(0.1mm)¡G\t0.000000\tVelocity(0.1mm0/s)¡G\t0.000000\tVoltage¡G\t-0.009766\nReal Periold(ms)¡G\t1\tEncoder Position(0.1mm)¡G\t0.000000\tVelocity(0.1mm0/s)¡G\t0.000000\tVoltage¡G\t0.003601\nReal Periold(ms)¡G\t1\tEncoder Position(0.1mm)¡G\t0.000000\tVelocity(0.1mm0/s)¡G\t0.000000\tVoltage¡G\t0.010284\nReal Periold(ms)¡G\t1\tEncoder Position(0.1mm)¡G\t0.000000\tVelocity(0.1mm0/s)¡G\t0.000000\tVoltage¡G\t0.005188\nReal Periold(ms)¡G\t1\tEncoder Position(0.1mm)¡G\t0.000000\tVelocity(0.1mm0/s)¡G\t0.000000\tVoltage¡G\t-0.001801\nReal Periold(ms)¡G\t1\tEncoder Position(0.1mm)¡G\t0.000000\tVelocity(0.1mm0/s)¡G\t0.000000\tVoltage¡G\t0.001068\nReal Periold(ms)¡G\t1\tEncoder Position(0.1mm)¡G\t0.000000\tVelocity(0.1mm0/s)¡G\t0.000000\tVoltage¡G\t0.009644\nReal Periold(ms)¡G\t1\tEncoder Position(0.1mm)¡G\t0.000000\tVelocity(0.1mm0/s)¡G\t0.000000\tVoltage¡G\t-0.011993\nReal Periold(ms)¡G\t1\tEncoder Position(0.1mm)¡G\t0.000000\tVelocity(0.1mm0/s)¡G\t0.000000\tVoltage¡G\t0.002014\nReal Periold(ms)¡G\t1\tEncoder Position(0.1mm)¡G\t0.000000\tVelocity(0.1mm0/s)¡G\t0.000000\tVoltage¡G\t-0.005310\nReal Periold(ms)¡G\t1\tEncoder Position(0.1mm)¡G\t0.000000\tVelocity(0.1mm0/s)¡G\t0.000000\tVoltage¡G\t-0.005615\nReal Periold(ms)¡G\t1\tEncoder Position(0.1mm)¡G\t0.000000\tVelocity(0.1mm0/s)¡G\t0.000000\tVoltage¡G\t-0.004028\nReal Periold(ms)¡G\t1\tEncoder Position(0.1mm)¡G\t0.000000\tVelocity(0.1mm0/s)¡G\t0.000000\tVoltage¡G\t0.001678\nReal Periold(ms)¡G\t1\tEncoder Position(0.1mm)¡G\t0.000000\tVelocity(0.1mm0/s)¡G\t0.000000\tVoltage¡G\t0.000427\nReal Periold(ms)¡G\t1\tEncoder Position(0.1mm)¡G\t0.000000\tVelocity(0.1mm0/s)¡G\t0.000000\tVoltage¡G\t0.009003\nReal Periold(ms)¡G\t1\tEncoder Position(0.1mm)¡G\t0.000000\tVelocity(0.1mm0/s)¡G\t0.000000\tVoltage¡G\t0.176117\nReal Periold(ms)¡G\t1\tEncoder Position(0.1mm)¡G\t0.000000\tVelocity(0.1mm0/s)¡G\t0.000000\tVoltage¡G\t0.004242\nReal Periold(ms)¡G\t1\tEncoder Position(0.1mm)¡G\t0.000000\tVelocity(0.1mm0/s)¡G\t0.000000\tVoltage¡G\t0.001678\nReal Periold(ms)¡G\t1\tEncoder Position(0.1mm)¡G\t0.000000\tVelocity(0.1mm0/s)¡G\t0.000000\tVoltage¡G\t0.003906\nReal Periold(ms)¡G\t1\tEncoder Position(0.1mm)¡G\t0.000000\tVelocity(0.1mm0/s)¡G\t0.000000\tVoltage¡G\t0.002319\nReal Periold(ms)¡G\t1\tEncoder Position(0.1mm)¡G\t0.000000\tVelocity(0.1mm0/s)¡G\t0.000000\tVoltage¡G\t0.000732\nReal Periold(ms)¡G\t1\tEncoder Position(0.1mm)¡G\t0.000000\tVelocity(0.1mm0/s)¡G\t0.000000\tVoltage¡G\t-0.008484\nReal Periold(ms)¡G\t1\tEncoder Position(0.1mm)¡G\t0.000000\tVelocity(0.1mm0/s)¡G\t0.000000\tVoltage¡G\t0.007111\nReal Periold(ms)¡G\t1\tEncoder Position(0.1mm)¡G\t0.000000\tVelocity(0.1mm0/s)¡G\t0.000000\tVoltage¡G\t-0.005615\nReal Periold(ms)¡G\t1\tEncoder Position(0.1mm)¡G\t0.000000\tVelocity(0.1mm0/s)¡G\t0.000000\tVoltage¡G\t0.015686\nReal Periold(ms)¡G\t1\tEncoder Position(0.1mm)¡G\t0.000000\tVelocity(0.1mm0/s)¡G\t0.000000\tVoltage¡G\t-0.003082\nReal Periold(ms)¡G\t1\tEncoder Position(0.1mm)¡G\t0.000000\tVelocity(0.1mm0/s)¡G\t0.000000\tVoltage¡G\t0.001373\nReal Periold(ms)¡G\t1\tEncoder Position(0.1mm)¡G\t0.000000\tVelocity(0.1mm0/s)¡G\t0.000000\tVoltage¡G\t0.002960\nReal Periold(ms)¡G\t1\tEncoder Position(0.1mm)¡G\t0.000000\tVelocity(0.1mm0/s)¡G\t0.000000\tVoltage¡G\t0.005188\nReal Periold(ms)¡G\t1\tEncoder Position(0.1mm)¡G\t0.000000\tVelocity(0.1mm0/s)¡G\t0.000000\tVoltage¡G\t-0.008484\nReal Periold(ms)¡G\t1\tEncoder Position(0.1mm)¡G\t0.000000\tVelocity(0.1mm0/s)¡G\t0.000000\tVoltage¡G\t0.000092\nReal Periold(ms)¡G\t1\tEncoder Position(0.1mm)¡G\t0.000000\tVelocity(0.1mm0/s)¡G\t0.000000\tVoltage¡G\t-0.008179\nReal Periold(ms)¡G\t1\tEncoder Position(0.1mm)¡G\t0.000000\tVelocity(0.1mm0/s)¡G\t0.000000\tVoltage¡G\t-0.000854\nReal Periold(ms)¡G\t1\tEncoder Position(0.1mm)¡G\t0.000000\tVelocity(0.1mm0/s)¡G\t0.000000\tVoltage¡G\t0.001678\nReal Periold(ms)¡G\t1\tEncoder Position(0.1mm)¡G\t0.000000\tVelocity(0.1mm0/s)¡G\t0.000000\tVoltage¡G\t0.000732\nReal Periold(ms)¡G\t1\tEncoder Position(0.1mm)¡G\t0.000000\tVelocity(0.1mm0/s)¡G\t0.000000\tVoltage¡G\t0.000092\nReal Periold(ms)¡G\t1\tEncoder Position(0.1mm)¡G\t0.000000\tVelocity(0.1mm0/s)¡G\t0.000000\tVoltage¡G\t0.001678\nReal Periold(ms)¡G\t1\tEncoder Position(0.1mm)¡G\t0.000000\tVelocity(0.1mm0/s)¡G\t0.000000\tVoltage¡G\t-0.019958\nReal Periold(ms)¡G\t1\tEncoder Position(0.1mm)¡G\t0.000000\tVelocity(0.1mm0/s)¡G\t0.000000\tVoltage¡G\t0.001373\nReal Periold(ms)¡G\t1\tEncoder Position(0.1mm)¡G\t0.000000\tVelocity(0.1mm0/s)¡G\t0.000000\tVoltage¡G\t-0.035217\nReal Periold(ms)¡G\t1\tEncoder Position(0.1mm)¡G\t0.000000\tVelocity(0.1mm0/s)¡G\t0.000000\tVoltage¡G\t0.007416\nReal Periold(ms)¡G\t1\tEncoder Position(0.1mm)¡G\t0.000000\tVelocity(0.1mm0/s)¡G\t0.000000\tVoltage¡G\t0.016022\nReal Periold(ms)¡G\t1\tEncoder Position(0.1mm)¡G\t0.000000\tVelocity(0.1mm0/s)¡G\t0.000000\tVoltage¡G\t-0.006897\nReal Periold(ms)¡G\t1\tEncoder Position(0.1mm)¡G\t0.000000\tVelocity(0.1mm0/s)¡G\t0.000000\tVoltage¡G\t0.009003\nReal Periold(ms)¡G\t1\tEncoder Position(0.1mm)¡G\t0.000000\tVelocity(0.1mm0/s)¡G\t0.000000\tVoltage¡G\t-0.010712\nReal Periold(ms)¡G\t1\tEncoder Position(0.1mm)¡G\t0.000000\tVelocity(0.1mm0/s)¡G\t0.000000\tVoltage¡G\t0.013794\nReal Periold(ms)¡G\t1\tEncoder Position(0.1mm)¡G\t0.000000\tVelocity(0.1mm0/s)¡G\t0.000000\tVoltage¡G\t-0.005951\nReal Periold(ms)¡G\t1\tEncoder Position(0.1mm)¡G\t0.000000\tVelocity(0.1mm0/s)¡G\t0.000000\tVoltage¡G\t-0.002777\nReal Periold(ms)¡G\t1\tEncoder Position(0.1mm)¡G\t0.000000\tVelocity(0.1mm0/s)¡G\t0.000000\tVoltage¡G\t-0.004028\nReal Periold(ms)¡G\t1\tEncoder Position(0.1mm)¡G\t0.000000\tVelocity(0.1mm0/s)¡G\t0.000000\tVoltage¡G\t-0.001160\nReal Periold(ms)¡G\t1\tEncoder Position(0.1mm)¡G\t0.000000\tVelocity(0.1mm0/s)¡G\t0.000000\tVoltage¡G\t-0.000549\nReal Periold(ms)¡G\t1\tEncoder Position(0.1mm)¡G\t0.000000\tVelocity(0.1mm0/s)¡G\t0.000000\tVoltage¡G\t0.012207\nReal Periold(ms)¡G\t1\tEncoder Position(0.1mm)¡G\t0.000000\tVelocity(0.1mm0/s)¡G\t0.000000\tVoltage¡G\t0.004547\nReal Periold(ms)¡G\t1\tEncoder Position(0.1mm)¡G\t0.000000\tVelocity(0.1mm0/s)¡G\t0.000000\tVoltage¡G\t-0.030151\nReal Periold(ms)¡G\t1\tEncoder Position(0.1mm)¡G\t0.000000\tVelocity(0.1mm0/s)¡G\t0.000000\tVoltage¡G\t-0.039368\nReal Periold(ms)¡G\t1\tEncoder Position(0.1mm)¡G\t0.000000\tVelocity(0.1mm0/s)¡G\t0.000000\tVoltage¡G\t-0.005310\nReal Periold(ms)¡G\t1\tEncoder Position(0.1mm)¡G\t0.000000\tVelocity(0.1mm0/s)¡G\t0.000000\tVoltage¡G\t-0.009460\nReal Periold(ms)¡G\t1\tEncoder Position(0.1mm)¡G\t0.000000\tVelocity(0.1mm0/s)¡G\t0.000000\tVoltage¡G\t-0.002441\nReal 
